vi "PZT capacity set.vi"(2 "error in (no error)":errorcluster caption="错误输入（无错误）", 3 "电容值（nF）":i32, 4 "VISA resource name":refnum<visa-resource-name> caption="VISA资源名称") -> (0 "错误输出":errorcluster, 1 "VISA资源名称输出":refnum<visa-resource-name>)   [LabVIEW 2019]
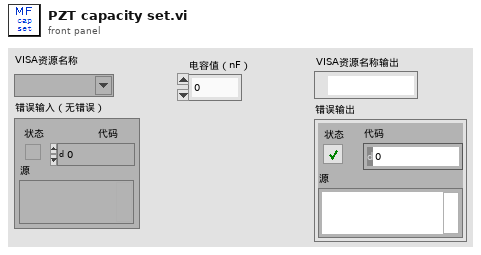
[diagram p1: front panel]
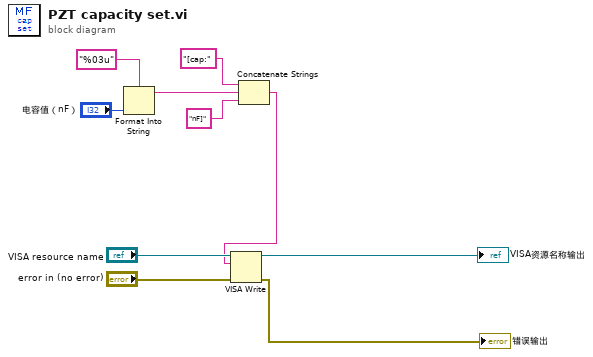
[diagram p0: block diagram]
diagram:
  n1 = Format Into String(format string="%03u" ("格式字符串"), "电容值（nF）") -> (resulting string=w5:string)  [unwired: 2 in, 1 out]
  n2 = Concatenate Strings("[cap:" ("字符串"), w5, "nF]" ("字符串")) -> (w2:string)
  n3 = VISA Write(VISA resource name="VISA resource name", write buffer=w2, error in (no error)="error in (no error)") -> (VISA resource name out=→"VISA资源名称输出":refnum<visa-resource-name>, error out=→"错误输出":errorcluster)  [unwired: 1 out]
